vi "Launch Dialog Box.vi"(7 "FP Window:Behavior (Floating)":T1(ring)=enum."Floating", 8 "error in (no error)":errorcluster, 9 "Auto-stop? (T)":bool=TRUE, 10 "DialogBox":refnum<class "IDialogBox.lvclass">, 11 "DialogBox Launcher":refnum<class "IViewable.lvclass">) -> (0 "error out":errorcluster, 2 "Dialog's Enqueuer":refnum<class "Message Enqueuer.lvclass">, 3 "DialogBox Launcher Out":refnum<class "IViewable.lvclass">)   [LabVIEW 2018, in "MVA Framework.lvlib" / "IDialogBox.lvlib" / "IDialogBox.lvclass"]
doc: "启动对话框"
uses:
  IDialogBox.lvclass
  <vilib>/ActorFramework/Actor/Actor.lvclass
  modules/mva-core/Source/IObserver/IObserver/IObserver.lvclass
  modules/mva-viewable/Source/IViewable/IViewable/IViewable.lvclass
  <vilib>/ActorFramework/Message Enqueuer/Message Enqueuer.lvclass
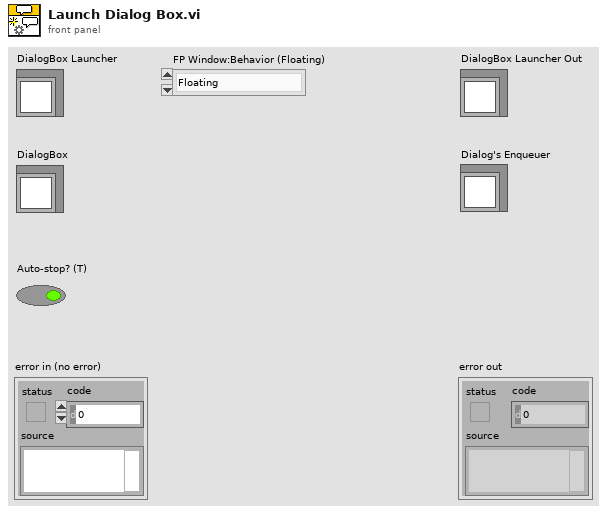
[diagram p1: front panel]
types:
  T1 = enum32{"Invalid", "Default", "Floating", "Floating/Auto-Hide", "Modal"}
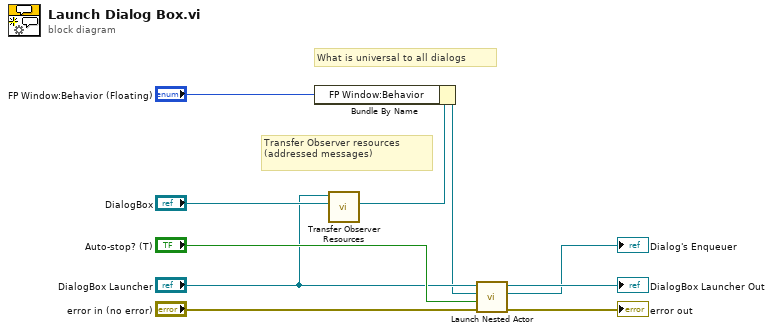
[diagram p0: block diagram]
diagram:
  # "Transfer Observer resources\n(addressed messages)"
  # "What is universal to all dialogs"
  n1 = call "Transfer Observer Resources.vi"("Recipient Observer In"="DialogBox", "Running Observer"="DialogBox Launcher") -> ("Recipient Observer Out"=w3:refnum<class "IDialogBox.lvclass">)  [unwired: 9 in]
  n2 = Bundle By Name(cluster=w3, "FP Window:Behavior"="FP Window:Behavior (Floating)") -> (w1:refnum<class "IDialogBox.lvclass">)
  n3 = call <vilib>:"Launch Nested Actor.vi"("error in (no error)"="error in (no error)", "Auto-stop? (T)"="Auto-stop? (T)", "Nested Actor"=w1, "Caller Actor in"="DialogBox Launcher") -> ("error out"=→"error out":errorcluster, "Nested Actor's Enqueuer"=→"Dialog's Enqueuer":refnum<class "Message Enqueuer.lvclass">, "Caller Actor out"=→"DialogBox Launcher Out":refnum<class "IViewable.lvclass">)  [unwired: 5 in]
